vi "loadMapping.vi"(8 "error in (no error)":errorcluster, 9 "xmlPath":string, 10 "channel_configXML":refnum<class "NativeXML.lvclass">, 11 "RfOutputChannel in":refnum<class "RfOutputChannel.lvclass">) -> (0 "error out":errorcluster, 3 "RfOutputChannel out":refnum<class "RfOutputChannel.lvclass">)   [LabVIEW 2009, in "Tools.lvlib" / "DatabaseHelpers.lvlib" / "RfOutputChannel.lvclass"]
uses:
  RfOutputChannel.lvclass
  NativeXML/NativeXML.lvclass
  RfOutputChannel.lvclass/RfOutputChannel.ctl
  Channel.lvclass
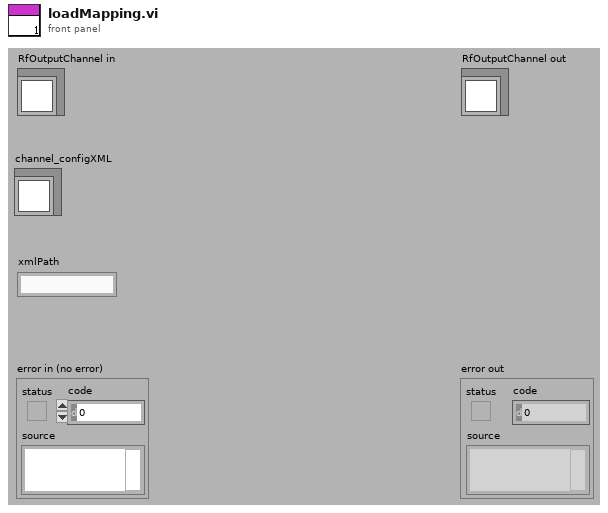
[diagram p1: front panel]
types:
  T1 = cluster{"Attribute String":string, "Value":string}
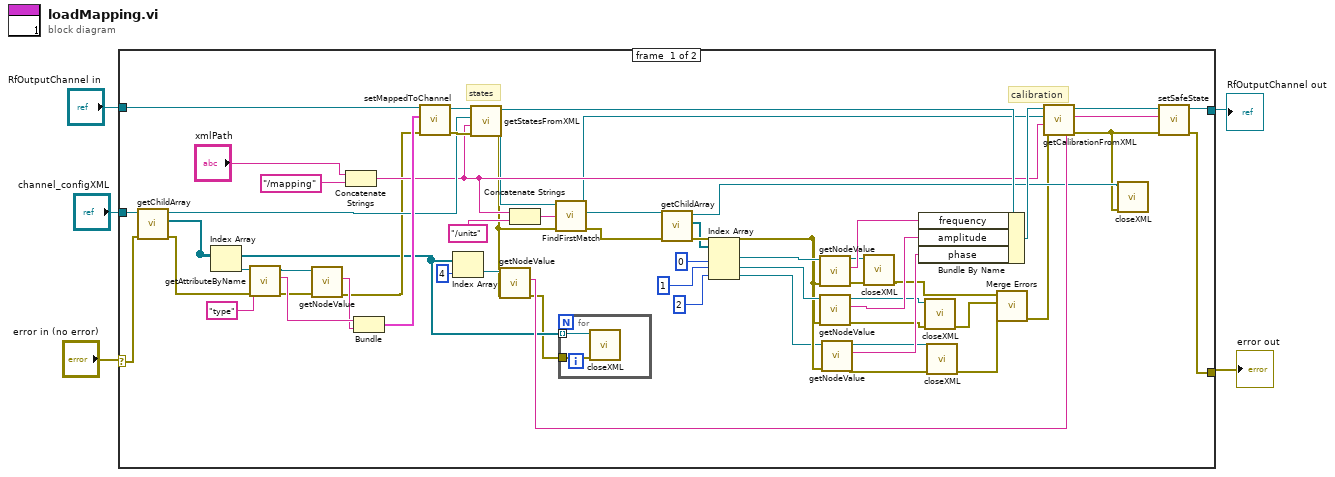
[diagram p0: block diagram]
diagram:
  n1 = case shown="No Error" "error in (no error)" {
    selector: "error in (no error)" -> [w49 w66]
    tunnel: [w54 w66] -> w5
    tunnel: [w55 w67] -> w2
    tunnel: "channel_configXML" -> [w50 _]
    tunnel: "RfOutputChannel in" -> [w58 w67]
    frame #0 {
      # "calibration"
      # "states"
      n2 = call "getChildArray.vi"("error in (no error)"=w49, "NativeXML in"=w50) -> ("error out"=w47:errorcluster, "childArray"=w7:refnum<class "NativeXML.lvclass">[], "NativeXML out"=w48:refnum<class "NativeXML.lvclass">)  [unwired: 7 in]
      n3 = Index Array(array=w7) -> (element=w46:refnum<class "NativeXML.lvclass">)  [unwired: 1 in]
      n4 = call "getAttributeByName.vi"("error in (no error)"=w47, "name"="type", "NativeXML in"=w46) -> ("error out"=w43:errorcluster, "Attribute String"=w44:string, "NativeXML out"=w42:refnum<class "NativeXML.lvclass">)  [unwired: 6 in]
      n5 = call "getNodeValue.vi"("error in (no error)"=w43, "NativeXML in"=w42) -> ("error out"=w8:errorcluster, "Value"=w41:string)  [unwired: 7 in, 1 out]
      n6 = Concatenate Strings("xmlPath", "/mapping") -> (w15:string)
      n7 = Bundle("Attribute String"=w44, "Value"=w41) -> (w60:T1)  [unwired: 1 in]
      n8 = call "setMappedToChannel.vi"("error in (no error)"=w8, "mappedTo"=w60, "Channel.lvclass in"=w58) -> ("error out"=w57:errorcluster, "Channel.lvclass out"=w59:refnum<class "RfOutputChannel.lvclass">)  [unwired: 7 in]
      n9 = Index Array(array=w7, index=4) -> (element=w40:refnum<class "NativeXML.lvclass">)
      n10 = call-dynamic "getStatesFromXML.vi"("error in (no error)"=w57, "xmlPath"=w15, "channel_configXML"=w48, "RfOutputChannel in"=w59) -> ("error out"=w13:errorcluster, "channel_configXML"=w14:refnum<class "NativeXML.lvclass">, "RfOutputChannel out"=w62:refnum<class "RfOutputChannel.lvclass">)  [unwired: 5 in]
      n11 = call "getNodeValue.vi"("error in (no error)"=w13, "NativeXML in"=w40) -> ("error out"=w6:errorcluster, "Value"=w39:string)  [unwired: 7 in, 1 out]
      n12 = Concatenate Strings(w15, "/units") -> (w9:string)
      n13 = call "FindFirstMatch.vi"("error in (no error)"=w13, "xPath"=w9, "NativeXML in"=w14) -> ("error out"=w12:errorcluster, "NativeXML match"=w10:refnum<class "NativeXML.lvclass">, "NativeXML out"=w11:refnum<class "NativeXML.lvclass">)  [unwired: 6 in]
      n14 = for {
        tunnel: w7 -> [w65] mode=indexing
        tunnel: w6 -> [w64]
        n15 = call "closeXML.vi"("error in (no error)"=w64, "NativeXML in"=w65) -> ()  [unwired: 9 in, 1 out]
      }
      n16 = call "getChildArray.vi"("error in (no error)"=w12, "NativeXML in"=w10) -> ("error out"=w34:errorcluster, "childArray"=w32:refnum<class "NativeXML.lvclass">[], "NativeXML out"=w31:refnum<class "NativeXML.lvclass">)  [unwired: 7 in]
      n17 = Index Array(array=w32, index #1=0, index #2=1, index #3=2) -> (element #1=w38:refnum<class "NativeXML.lvclass">, element #2=w36:refnum<class "NativeXML.lvclass">, element #3=w33:refnum<class "NativeXML.lvclass">)
      n18 = call "getNodeValue.vi"("error in (no error)"=w34, "NativeXML in"=w38) -> ("error out"=w27:errorcluster, "Value"=w29:string, "NativeXML out"=w28:refnum<class "NativeXML.lvclass">)  [unwired: 7 in]
      n19 = call "getNodeValue.vi"("error in (no error)"=w34, "NativeXML in"=w36) -> ("error out"=w25:errorcluster, "Value"=w37:string, "NativeXML out"=w24:refnum<class "NativeXML.lvclass">)  [unwired: 7 in]
      n20 = call "getNodeValue.vi"("error in (no error)"=w34, "NativeXML in"=w33) -> ("error out"=w21:errorcluster, "Value"=w35:string, "NativeXML out"=w20:refnum<class "NativeXML.lvclass">)  [unwired: 7 in]
      n21 = call "closeXML.vi"("error in (no error)"=w27, "NativeXML in"=w28) -> ("error out"=w26:errorcluster)  [unwired: 9 in]
      n22 = Bundle By Name(cluster=w62, "frequency"=w29, "amplitude"=w37, "phase"=w35) -> (w61:refnum<class "RfOutputChannel.lvclass">)
      n23 = call "closeXML.vi"("error in (no error)"=w25, "NativeXML in"=w24) -> ("error out"=w23:errorcluster)  [unwired: 9 in]
      n24 = call "closeXML.vi"("error in (no error)"=w21, "NativeXML in"=w20) -> ("error out"=w22:errorcluster)  [unwired: 9 in]
      n25 = call <vilib>:"Merge Errors.vi"("error in 3 (no error)"=w22, "error in 2 (no error)"=w23, "error in 1 (no error)"=w26) -> ("error out"=w30:errorcluster)  [unwired: 4 in]
      n26 = call-dynamic "getCalibrationFromXML.vi"("error in (no error)"=w30, "xmlPath"=w15, "channel_configXML"=w11, "RfOutputChannel in"=w61) -> ("error out"=w19:errorcluster, "RfOutputChannel out"=w56:refnum<class "RfOutputChannel.lvclass">)  [unwired: 5 in, 1 out]
      n27 = call "closeXML.vi"("error in (no error)"=w19, "NativeXML in"=w31) -> ()  [unwired: 9 in, 1 out]
      n28 = call "setSafeState.vi"("error in (no error)"=w19, "safe_state"=w39, "Channel.lvclass in"=w56) -> ("error out"=w54:errorcluster, "Channel.lvclass out"=w55:refnum<class "RfOutputChannel.lvclass">)  [unwired: 7 in]
    }
    frame #1 {
    }
  }
  "error out" <- w5
  "RfOutputChannel out" <- w2
